vi "SetMemory_byPtr.vi"(5 "error in (no error)":errorcluster, 7 "Input":string, 8 "Pointer":i32) -> (0 "error out":errorcluster, 3 "Duplicate Pointer":i32)   [LabVIEW 2011]
doc: "This VI sets memory on the heap beginning at the address specified by <B>Pointer</B>. The VI requires data to be written as a flattened data string."
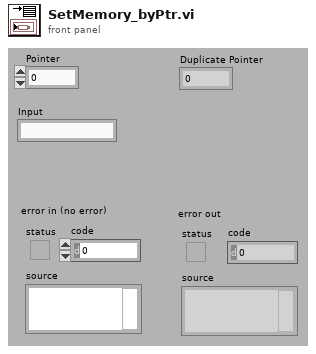
[diagram p1: front panel]
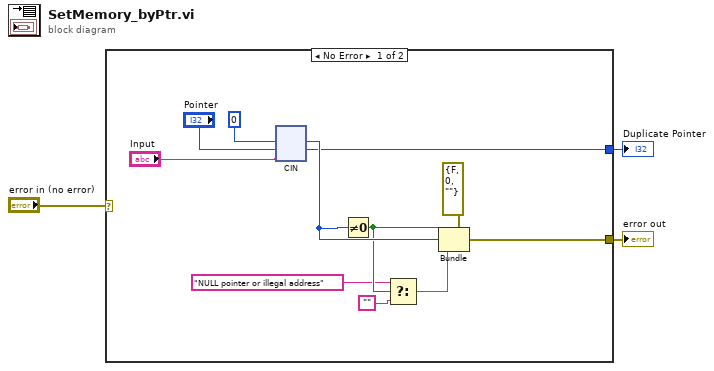
[diagram p0: block diagram]
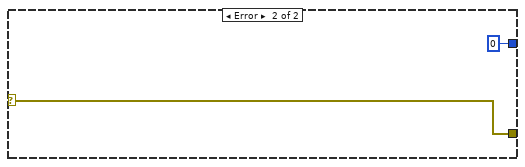
[diagram p2: hidden frame]
diagram:
  n1 = case shown="No Error" "error in (no error)" {
    selector: "error in (no error)" -> [_ w16]
    tunnel: [w13 w16] -> w2
    tunnel: [w9 0 ("Pointer")] -> w1
    frame No Error {
      n2 = cin(0, "Pointer", "Input") -> (w10:i32, w9:i32)  [unwired: 1 in]
      n3 = Not Equal To 0?(x=w10) -> (x != 0?=w8:bool)
      n4 = Select(t="NULL pointer or illegal address", s=w8, f="") -> (s? t:f=w6:string)
      n5 = Bundle(cluster=errorcluster {"status"=FALSE, "code"=0, "source"=""} ("error in (no error)"), "status"=w8, "code"=w10, "source"=w6) -> (w13:errorcluster)
    }
    frame Error {
    }
  }
  "error out" <- w2
  "Duplicate Pointer" <- w1
